vi "Write Reset.vi"(8 "error in":errorcluster, 10 "Reset Arguments":T1=enum."Reset counter (all)", 11 "MB_TCP session in":refnum<class "MB_Master_TCP.lvclass">) -> (0 "error out":errorcluster, 3 "MB session out":refnum<class "MB_Master_TCP.lvclass">)   [LabVIEW 2024, in "Bronkhorst Flexi-Flow ModbusTCP API.lvlib"]
uses:
  Bronkhorst Flexi-Flow ModbusTCP API.lvlib
  <vilib>/Plasmionique/MB Master/MB_Master_TCP/MB_Master_TCP.lvclass
  Reset Counter--enum.ctl
  PDU Address Char 8-bit Params--ring.ctl
  Write Unsigned Int Register.vi
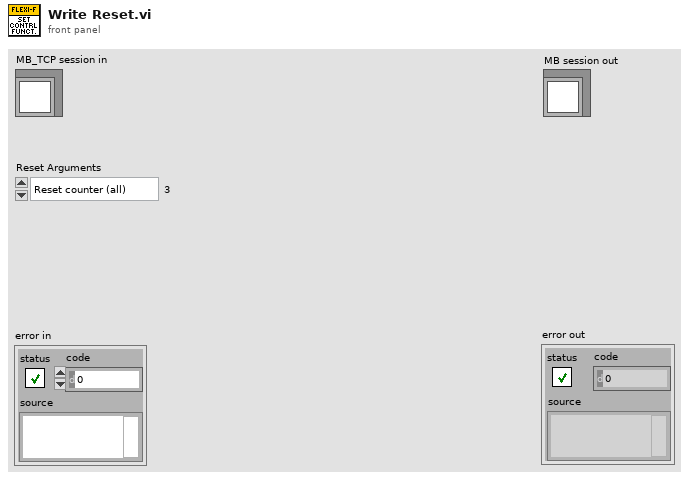
[diagram p1: front panel]
types:
  T1 = typedef "Bronkhorst Flexi-Flow ModbusTCP API.lvlib/Reset Counter--enum.ctl" = enum16{"No reset", "Reset counter", "Reset alarm", "Reset counter (all)", "Reset and disable counter", "Reset firmware program (soft reset)", "Reset Alarm infor error bit", "Reset Alarm info warning bit"}
  T2 = typedef "Bronkhorst Flexi-Flow ModbusTCP API.lvlib/PDU Address Char 8-bit Params--ring.ctl" = u16
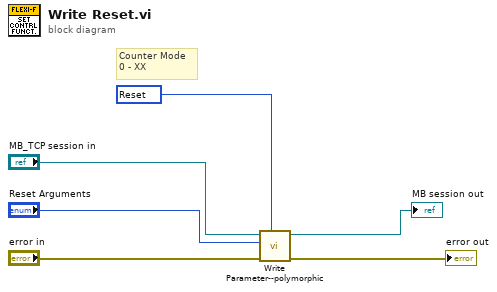
[diagram p0: block diagram]
diagram:
  w4 = T2 3688 items=["Wink"=0, "Control mode"=36, "Alarm mode"=3107, "Alarm setpoint"=3109, "Reset alarm enable"=3113, "Counter unit index"=3330, "Counter setpoint mode"=3333, "Counter mode"=3336, "Reset counter enable"=3337, "Reset"=3688, "Modbus slave address"=4010] ("PDU Address Char 8-bit")
  # "Counter Mode\n0 - XX"
  n1 = call-poly "Write Parameter--polymorphic.vi"("PDU Address (U-Int16)"=w4, "error in"="error in", "Value"="Reset Arguments", "MB_TCP session in"="MB_TCP session in") -> ("error out"=→"error out":errorcluster, "MB session out"=→"MB session out":refnum<class "MB_Master_TCP.lvclass">)  [unwired: 6 in]
